vi "VecBuilder_4x1Fill.vi"(8 "R3":dbl, 9 "R2":dbl, 10 "R1":dbl, 11 "R0":dbl) -> (3 "output matrix":T1)   [LabVIEW 2019, in "Trajectory_Library.lvlib"]
doc: "Creates a new LINEAR SYSTEM data cluster with the specified values. \n\n\nInputs: \n - XXX -- XXX.\n\nOutputs:\n - XXX -- XXX."
uses:
  Trajectory_Library.lvlib
  <vilib>/Analysis/Matrix/Datatypes/RealMatrix.ctl
  <vilib>/Analysis/Matrix/NI_Matrix.lvlib
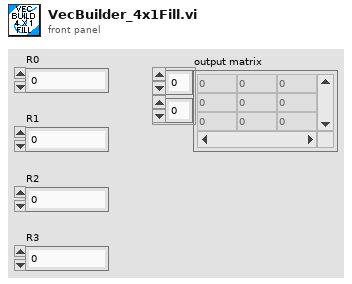
[diagram p1: front panel]
types:
  T1 = typedef "NI_Matrix.lvlib/RealMatrix.ctl" = dbl[][]
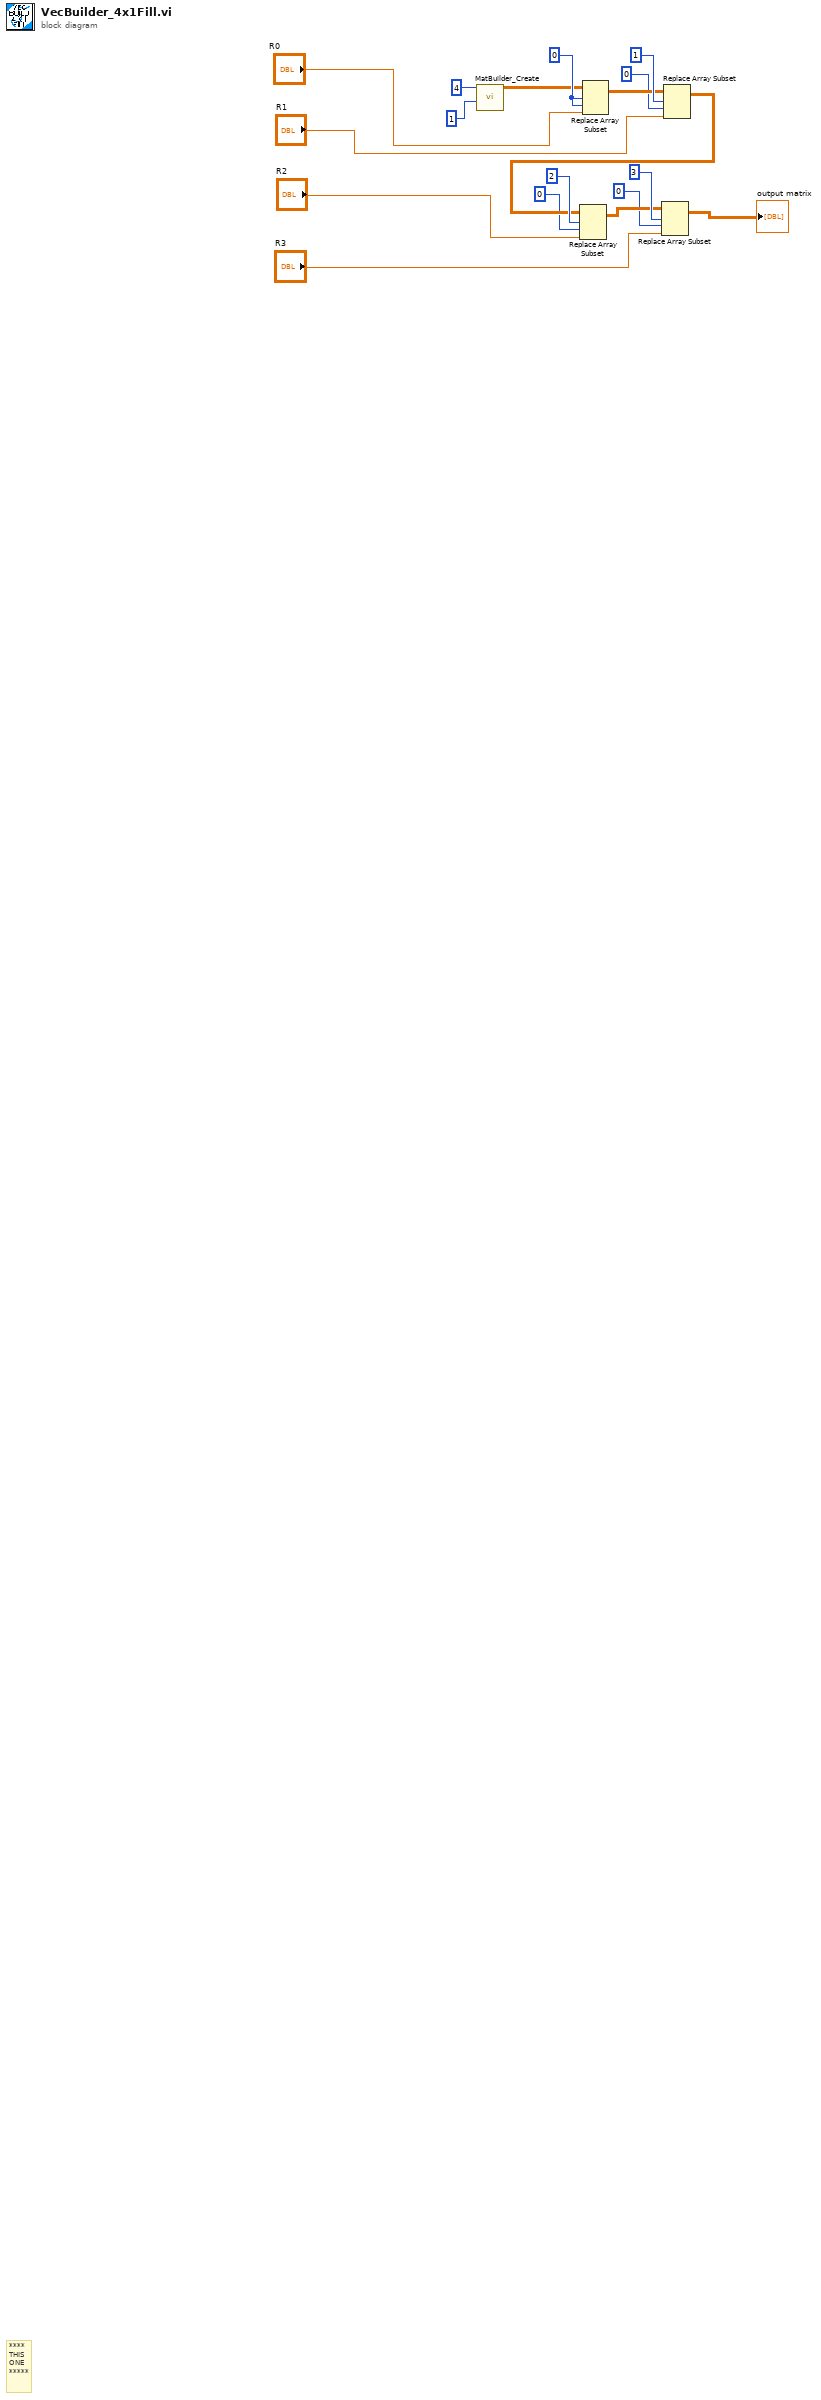
[diagram p0: block diagram]
diagram:
  w18 = 0 ("index (col)")
  # "****\nTHIS\nONE\n*****"
  n1 = call "MatBuilder_Create.vi"("Columns"=1, "Rows"=4) -> ("output matrix"=w10:T1)  [unwired: 9 in]
  n2 = Replace Array Subset(array=w10, new element="R0", index (row)=w18, index (col)=w18) -> (w16:T1)
  n3 = Replace Array Subset(array=w16, new element="R1", index (row)=1 ("index (col)"), index (col)=0 ("disabled index (col)")) -> (w7:T1)
  n4 = Replace Array Subset(array=w7, new element="R2", index (row)=2 ("index (col)"), index (col)=0 ("disabled index (col)")) -> (w6:T1)
  n5 = Replace Array Subset(array=w6, new element="R3", index (row)=3 ("index (col)"), index (col)=0 ("disabled index (col)")) -> (→"output matrix":T1)
